vi "Target.vi"() -> ()   [LabVIEW 2017]
uses:
  Controls/Outputs.ctl
  <vilib>/Platform/TimedLoop/XDataNode/timing_clust.ctl
  <vilib>/Platform/TimedLoop/XDataNode/nitl_modes.ctl
  <vilib>/Platform/TimedLoop/XDataNode/wakeup.ctl
  <vilib>/myRIO/Instrument Drivers/Onboard IO/PWM/typedefs/PWM Reference.ctl
  <vilib>/myRIO/Common/Instrument Driver Framework/Utilities/typedefs/myRIO Generic Hardware Reference.ctl
  <vilib>/myRIO/Common/Instrument Driver Framework/Utilities/typedefs/Hardware Version Enum.ctl
  <vilib>/myRIO/Common/Instrument Driver Framework/Utilities/typedefs/myRIO v1.0 Reference.ctl
  <vilib>/myRIO/Common/Instrument Driver Framework/Utilities/typedefs/Generic FPGA Reference.ctl
  <vilib>/myRIO/Common/Instrument Driver Framework/myRIO v1.0/PWM/typedefs/PWM Channels Enum.ctl
  <vilib>/myRIO/Instrument Drivers/Onboard IO/PWM/typedefs/PWM Configuration.ctl
  <vilib>/userdefined/High Color/nirio_resource_hc.ctl
  <vilib>/myRIO/Instrument Drivers/Onboard IO/DIO/typedefs/DIO Reference.ctl
  <vilib>/myRIO/Common/Instrument Driver Framework/myRIO v1.0/DIO/typedefs/DIO Channels List.ctl
  <vilib>/myRIO/Common/Instrument Driver Framework/myRIO v1.0/DIO/typedefs/DIO Channels Enum.ctl
  <vilib>/myRIO/Common/Instrument Driver Framework/Utilities/vis/Is FPGA Ref Available.vi
  <vilib>/myRIO/Common/Instrument Driver Framework/myRIO v1.0/PWM/vis/myRIO v1.1 Open PWM.vi
  <vilib>/myRIO/Instrument Drivers/Onboard IO/PWM/vis/Set Duty Cycle and Frequency.vi
  <vilib>/myRIO/Common/Instrument Driver Framework/myRIO v1.0/DIO/vis/myRIO v1.1 Open DIO.vi
  <extravilib>/ChannelInstances/Tag-dbl/Read With Abort.vi
  <vilib>/myRIO/Common/Instrument Driver Framework/Utilities/vis/Validate Channels.vi
  <vilib>/myRIO/Common/Instrument Driver Framework/myRIO v1.0/PWM/vis/myRIO v1.0 Reserve PWM.vi
  <vilib>/myRIO/Common/Instrument Driver Framework/myRIO v1.0/DIO/vis/myRIO v1.0 Reserve DIO.vi
  <extravilib>/ChannelInstances/Tag-dbl/Write With Abort.vi
  <vilib>/myRIO/Common/Instrument Driver Framework/myRIO v1.0/UART/vis/myRIO v1.0 Close UART.vi
  <vilib>/myRIO/Common/Instrument Driver Framework/myRIO v1.0/PWM/vis/myRIO v1.0 Build MUX Configuration PWM.vi
  <vilib>/myRIO/Common/Instrument Driver Framework/myRIO v1.0/Resource Manager/vis/myRIO v1.0 Reserve Channel List.vi
  <vilib>/myRIO/Common/Instrument Driver Framework/myRIO v1.0/DIO/vis/myRIO v1.0 Build MUX Configuration DIO.vi
  <vilib>/myRIO/Common/Instrument Driver Framework/myRIO v1.0/Resource Manager/vis/myRIO v1.0 Create Configuration List.vi
  <vilib>/myRIO/Common/Instrument Driver Framework/myRIO v1.0/Resource Manager/vis/myRIO v1.0 Reserve Channel.vi
  <vilib>/myRIO/Common/Instrument Driver Framework/myRIO v1.0/Resource Manager/vis/myRIO v1.0 Unreserve Channel.vi
  <vilib>/myRIO/Common/Instrument Driver Framework/myRIO v1.0/Resource Manager/vis/myRIO v1.0 Build Mutex Name.vi
  <vilib>/Utility/VariantDataType/GetNumericInfo.vi
  <vilib>/Utility/error.llb/Error Cluster From Error Code.vi
  <vilib>/myRIO/Common/Instrument Driver Framework/myRIO v1.0/myRIO v1.1 Open.vi
  <vilib>/myRIO/Common/Instrument Driver Framework/Utilities/vis/IO Manager.vi
  <vilib>/myRIO/Common/Instrument Driver Framework/Utilities/vis/Configuration Manager.vi
  <vilib>/myRIO/Common/Instrument Driver Framework/myRIO v1.0/Resource Manager/vis/myRIO v1.0 Configure IO.vi
  <vilib>/myRIO/Common/Instrument Driver Framework/myRIO v1.0/myRIO v1.0 Close.vi
  <vilib>/myRIO/Common/Instrument Driver Framework/myRIO v1.0/DIO/vis/myRIO v1.0 Write DIO.vi
  <extravilib>/ChannelInstances/Tag-dbl/Instantiate.vi
  <extravilib>/ChannelInstances/Tag-dbl/EndpointRead.vi
  <vilib>/myRIO/Common/Instrument Driver Framework/myRIO v1.0/PWM/vis/myRIO v1.0 Write PWM.vi
  <extravilib>/ChannelInstances/Tag-dbl/Endpoint.vi
  <vilib>/myRIO/Common/Instrument Driver Framework/Utilities/vis/FPGA Ref Manager.vi
  <vilib>/myRIO/Common/Instrument Driver Framework/myRIO v1.0/myRIO v1.0 Reset FPGA.vi
  <vilib>/myRIO/Common/Instrument Driver Framework/myRIO v1.0/IRQ/vis/myRIO v1.0 IRQ Info FGV.vi
  <vilib>/myRIO/Common/Instrument Driver Framework/myRIO v1.0/IRQ/vis/myRIO v1.0 Timer IRQ Info FGV.vi
  <vilib>/myRIO/Common/Instrument Driver Framework/myRIO v1.0/IRQ/vis/myRIO v1.0 ISR Agent.vi
  <vilib>/Platform/TimedLoop/XDataNode/XDataNode.xnode
  <vilib>/myRIO/Express VI/Onboard IO/DO/DO Express VI.xnode
  <vilib>/myRIO/Instrument Drivers/Onboard IO/DIO/vis/myRIO DIO Open.xnode
  <vilib>/myRIO/Express VI/Onboard IO/PWM/PWM Express VI.xnode
  <vilib>/myRIO/Instrument Drivers/Onboard IO/PWM/vis/myRIO PWM Open.xnode
  <vilib>/myRIO/Instrument Drivers/Utilities/Utilities.lvlib
  <vilib>/Platform/TimedLoop/XDataNode/XDNodeRunTimeDep.lvlib
  <vilib>/myRIO/Instrument Drivers/Onboard IO/PWM/PWM.lvlib
  <vilib>/myRIO/Instrument Drivers/Onboard IO/DIO/DIO.lvlib
  <extravilib>/ChannelInstances/Tag-dbl.lvlib
panel:
  out "StateData 2":T1
  out "Cup Data":T2
  out "Boolean":bool
  out "Outputs":T3
  out "Duty Cycle Top Indicator":dbl=0.8
  out "Duty Cycle Base Indicator":dbl=0.8
  out "theta":dbl
  out "phi":dbl
  out "Iteration Duration":i64
  in  "stop":bool
  out "Target Running":bool
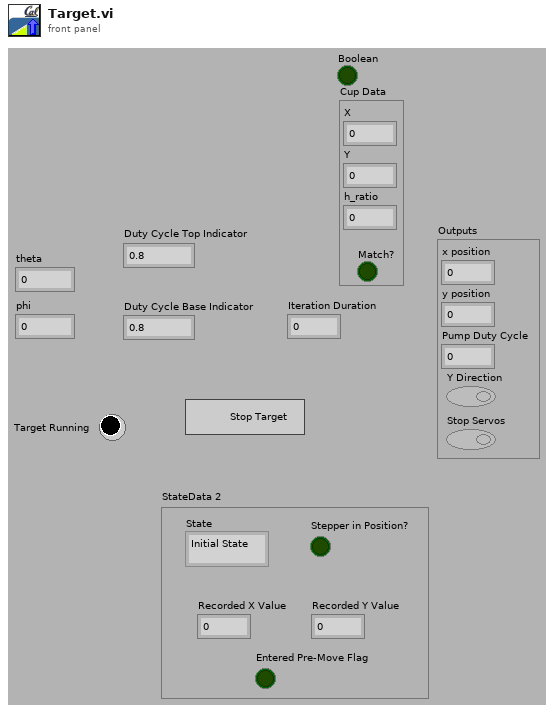
[diagram p1: front panel]
types:
  T1 = cluster{"State":enum16{"Initial State", "Pre Move", "Move Arm", "Fill Water"}, "Stepper in Position?":bool, "Recorded X Value":dbl, "Recorded Y Value":dbl, "Entered Pre-Move Flag":bool}
  T2 = cluster{"X":dbl, "Y":dbl, "h_ratio":dbl, "Match?":bool}
  T3 = typedef "Outputs.ctl" = cluster{"x position":dbl, "y position":dbl, "Pump Duty Cycle":dbl, "Y Direction":bool, "Stop Servos":bool}
  T4 = typedef "XDNodeRunTimeDep.lvlib/timing_clust.ctl" = cluster{"Expected End [f-1]":u64, "Actual End [f-1]":u64, "Finished Late? [f-1]":bool, "Expected End [i-1]":u64, "Actual End [i-1]":u64, "Finished Late? [i-1]":bool, "Expected Start [i]":u64, "Actual Start [i]":u64, "Expected Start [f]":u64, "Actual Start [f]":u64, "Source Name":string, "Structure Name":string, "Period":i64, "Deadline":i64, "Offset":i64, "Start":i64, "Priority":i32, "Timeout":i32, "Mode":T5, "Wakeup Reason":T6, "Error":errorcluster, "Source Type":string, "Secondary Source Type":string, "Global End Time":u64, "Global Start Time":u64, "Frame Duration":u64, "Iteration Duration":u64, "Assigned CPU":i32, "I/O Scan Engine Mode":u32}
  T5 = typedef "XDNodeRunTimeDep.lvlib/nitl_modes.ctl" = enum32{"No Change", "Process missed periods, maintain original phase", "Discard missed periods, maintain original phase", "Process missed periods, ignore original phase", "Discard missed periods, ignore original phase"}
  T6 = typedef "XDNodeRunTimeDep.lvlib/wakeup.ctl" = enum32{"Normal", "Aborted", "Asynchronous wakeup", "Timing source error", "Timed loop error", "Timeout"}
  T7 = typedef "PWM.lvlib/PWM Reference.ctl" = cluster{"myRIO Reference":T8, "PWM Channels Enum":T12, "PWM Configuration":T13}
  T8 = typedef "myRIO Generic Hardware Reference.ctl" = cluster{"myRIO Model":T9, "myRIO Hardware Reference":T10}
  T9 = typedef "Hardware Version Enum.ctl" = enum16{"Unknown", "myRIO-1900", "myRIO-1950", "roboRIO", "NI ELVIS RIO CM"}
  T10 = typedef "myRIO v1.0 Reference.ctl" = cluster{"Generic FPGA Reference":T11, "Allow multiple opens":bool}
  T11 = typedef "Generic FPGA Reference.ctl" = refnum<k20>
  T12 = typedef "PWM Channels Enum.ctl" = enum16{"Not Connected", "C/PWM0", "C/PWM1", "A/PWM0", "A/PWM1", "A/PWM2", "B/PWM0", "B/PWM1", "B/PWM2", "PWM/PWM0", "PWM/PWM1", "PWM/PWM2", "PWM/PWM3", "PWM/PWM4", "PWM/PWM5", "PWM/PWM6", "PWM/PWM7", "PWM/PWM8", "PWM/PWM9"}
  T13 = typedef "PWM.lvlib/PWM Configuration.ctl" = cluster{"Frequency":dbl, "Duty Cycle":dbl}
  T14 = typedef "nirio_resource_hc.ctl" = tag
  T15 = typedef "Tag-dbl.lvlib/))Channel.ctl" = refnum<queue>
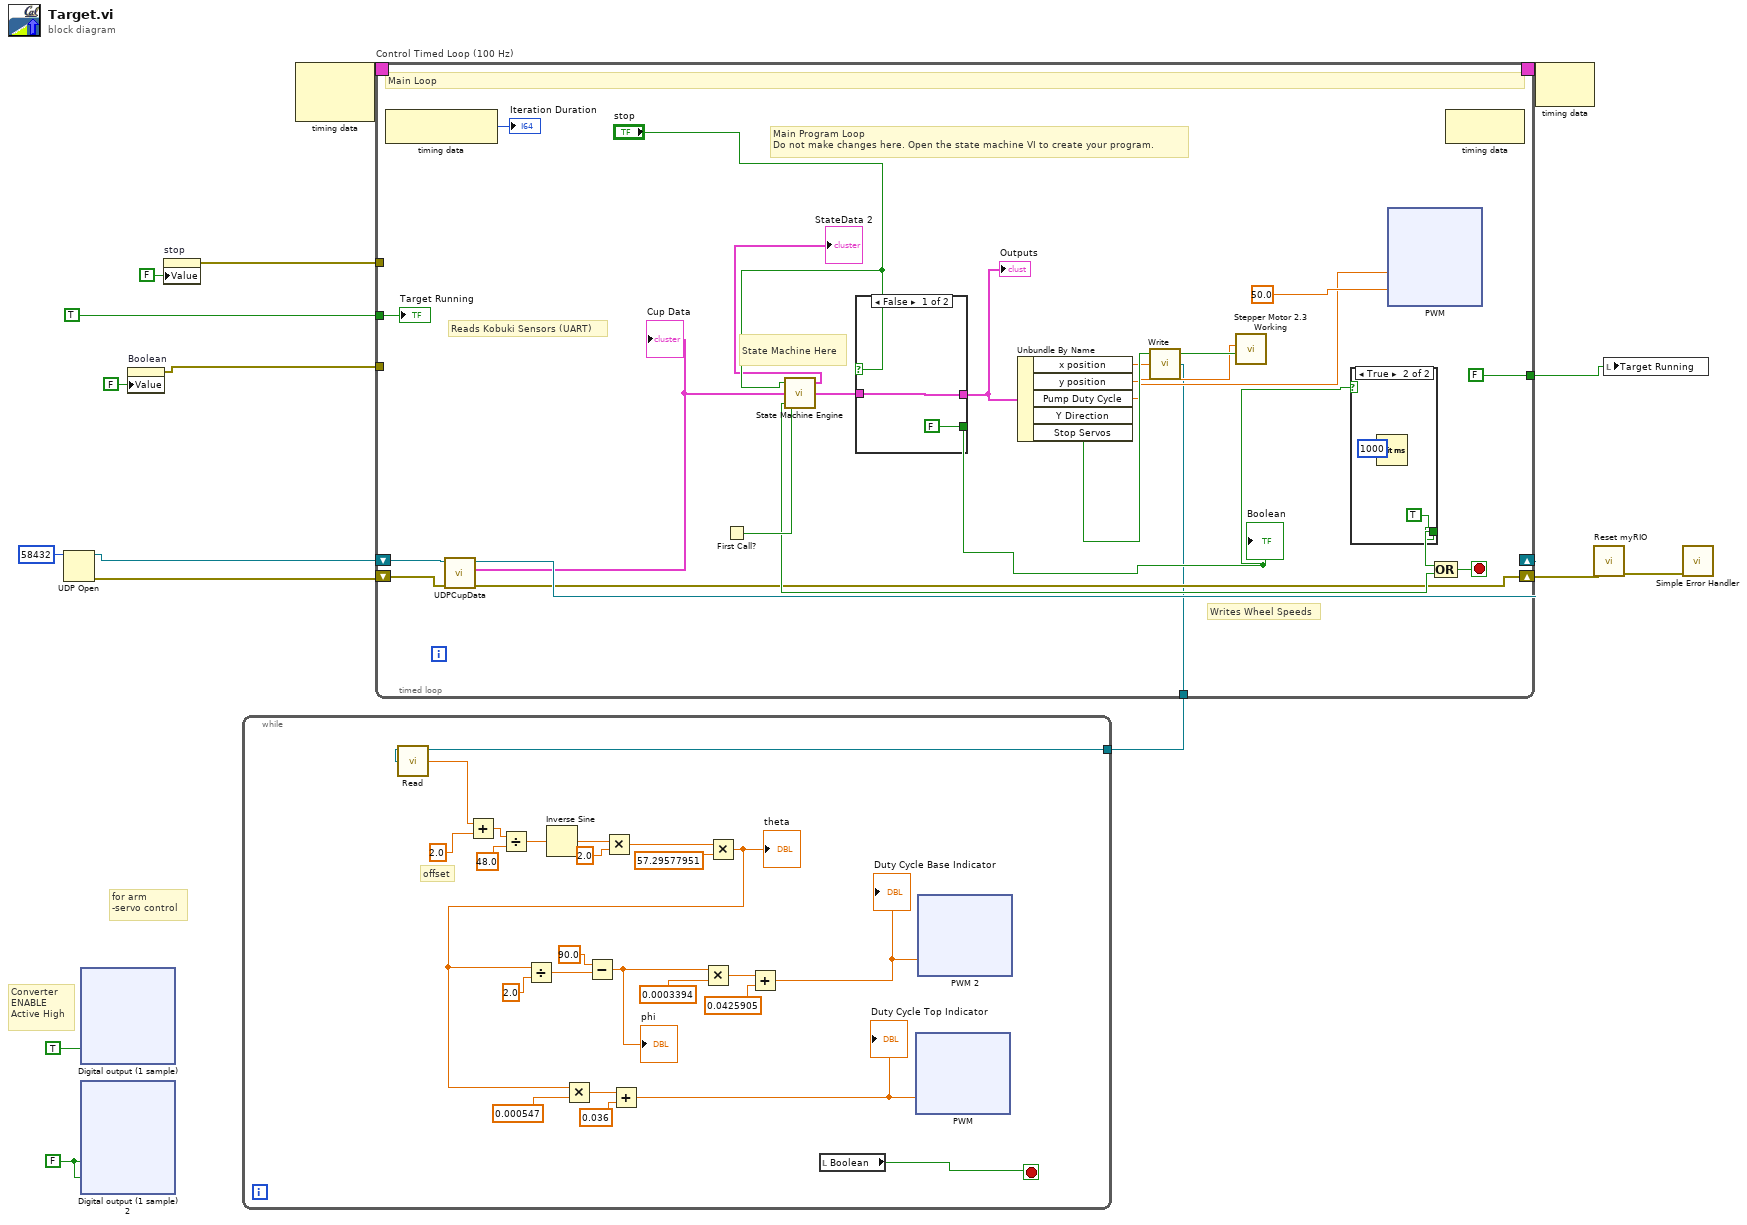
[diagram p0: block diagram]
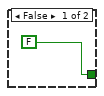
[diagram p2: hidden frame]
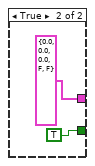
[diagram p3: hidden frame]
diagram:
  w6 = FALSE
  # "for arm\n-servo control"
  # "Converter\nENABLE\nActive High"
  n1 = UDP Open(11:u16 58432 ("port")) -> (port=w9:refnum<k16>, 0:w10:errorcluster)  [unwired: 4 in, 1 out]
  n2 = xnode "Digital output (1 sample)"("B/DIO4 (Pin 19)"=TRUE) -> ()  [unwired: 1 in, 1 out]
  n3 = xnode "Digital output (1 sample) 2"("B/DIO3 (Pin 17)"=w6, "B/DIO1 (Pin 13)"=w6) -> ()  [unwired: 1 in, 1 out]
  n4 = property on="Boolean" class="Bool (strict)"("Value"=FALSE ("Boolean")) -> (error out=w4:errorcluster)  [unwired: 2 in, 1 out]
  n5 = property on="stop" class="Bool (strict)"("Value"=FALSE ("stop")) -> (error out=w2:errorcluster)  [unwired: 2 in, 1 out]
  n6 = node-c288() -> (w13:T4)  [unwired: 2 in]
  n7 = timed-loop "Control Timed Loop (100 Hz)" {
    shift-right: [w26] -> w8
    shift-left: w10 -> [w32]
    tunnel: TRUE ("stop") -> [w37]
    tunnel: [FALSE ("stop")] -> w15
    timing: w13 -> [_]
    timing-out: [_] -> w12
    shift-right: [w30] -> _
    shift-left: w9 -> [w31]
    tunnel: w4 -> [_]
    tunnel: w2 -> [_]
    tunnel: [w18] -> w1
    stop <- w39 stop-if-true
    # "Main Program Loop\nDo not make changes here. Open the state machine VI to create your program."
    # "Writes Wheel Speeds"
    # "Reads Kobuki Sensors (UART)"
    # "State Machine Here"
    # "Main Loop"
    n8 = node-c288() -> (→"Iteration Duration":i64)  [unwired: 1 in]
    n9 = call "UDPCupData.vi"("error in (no error)"=w32, "UDP Network Connection in"=w31) -> ("error out"=w26:errorcluster, "Cup Data"=w29:T2, "UDP Network Connection out"=w30:refnum<k16>)  [unwired: 7 in]
    "Cup Data" <- w29
    n10 = First Call?() -> (First Call?: T/F=w36:bool)
    n11 = call "State Machine Engine.vi"("Init?"=w36, "Inputs"=w29, "Stop"="stop") -> ("Terminated?"=w35:bool, "Outputs"=w23:T3, "StateData"=→"StateData 2":T1)
    n12 = case shown="False" "stop" {
      tunnel: [w44 T3 {"x position"=0.0, "y position"=0.0, "Pump Duty Cycle"=0.0, "Y Direction"=FALSE, "Stop Servos"=FALSE} ("Outputs")] -> w24
      tunnel: w23 -> [w44 _]
      tunnel: [FALSE TRUE] -> w20
      frame False {
      }
      frame True {
      }
    }
    "Outputs" <- w24
    "Boolean" <- w20
    n13 = Unbundle By Name(w24) -> ("x position"=w19:dbl, "y position"=w25:dbl, "Pump Duty Cycle"=w27:dbl, "Y Direction"=w28:bool)  [unwired: 1 out]
    n14 = call <extravilib>:"Write.vi"("element"=w19) -> ("channel"=w18:T15)  [unwired: 1 out]
    n15 = call "Stepper Motor 2.3 Working.vi"("Dir"=w28, "y (inches)"=w25) -> ()  [unwired: 10 in]
    n16 = case shown="True" w20 {
      tunnel: [FALSE ("stop") TRUE] -> w21
      frame False {
      }
      frame True {
        n17 = Wait (ms)(milliseconds to wait=u32 1000) -> ()  [unwired: 1 out]
      }
    }
    n18 = xnode "PWM"("Duty Cycle"=w27, "Frequency [Hz]"=50.0) -> ()  [unwired: 1 in, 1 out]
    n19 = Compound Arithmetic op=OR(w21, w35) -> (w39:bool)
    n20 = node-c288() -> ()  [unwired: 1 in, 1 out]
    "Target Running" <- w37
  }
  n21 = while {
    tunnel: w1 -> [w86]
    stop <- w87 stop-if-true
    # "offset"
    n22 = call <extravilib>:"Read.vi"("channel"=w86) -> ("element"=w85:dbl)  [unwired: 1 in, 1 out]
    n23 = Add(x=w85, y=2.0) -> (x+y=w88:dbl)
    n24 = Divide(x=w88, y=48.0) -> (x/y=w107:dbl)
    n25 = Inverse Sine(1:w107) -> (0:w105:dbl)
    n26 = Multiply(x=w105, y=2.0) -> (x*y=w102:dbl)
    n27 = Multiply(x=w102, y=57.29577951) -> (x*y=w93:dbl)
    "theta" <- w93
    n28 = Divide(x=w93, y=2.0) -> (x/y=w104:dbl)
    n29 = Multiply(x=w93, y=0.000547) -> (x*y=w100:dbl)
    n30 = Subtract(x=90.0, y=w104) -> (x-y=w92:dbl)
    "phi" <- w92
    n31 = Add(x=w100, y=0.036) -> (x+y=w90:dbl)
    "Duty Cycle Top Indicator" <- w90
    n32 = Multiply(x=w92, y=0.0003394) -> (x*y=w97:dbl)
    n33 = Add(x=w97, y=0.0425905) -> (x+y=w91:dbl)
    "Duty Cycle Base Indicator" <- w91
    n34 = local read "Boolean"() -> (w87:bool)
    n35 = xnode "PWM"("Duty Cycle"=w90) -> ()  [unwired: 1 in, 1 out]
    n36 = xnode "PWM 2"("Duty Cycle"=w91) -> ()  [unwired: 1 in, 1 out]
  }
  n37 = node-c288(w12) -> ()  [unwired: 1 out]
  n38 = call <vilib>:"Reset myRIO.vi"("error in (no error)"=w8) -> ("error out"=w14:errorcluster)  [unwired: 10 in]
  n39 = local write "Target Running"(w15) -> ()
  n40 = call <vilib>:"Simple Error Handler.vi"("error in (no error)"=w14) -> ()  [unwired: 4 in, 5 out]
